vi "Get Path Commands.vi"(1 "Commands Raw Data":string) -> (0 "Array of Commands":T1(array[cluster]))   [LabVIEW 2011]
doc: "This VI takes in raw path data and outputs an array of all the commands found."
uses:
  <vilib>/Utility/error.llb/whitespace.ctl
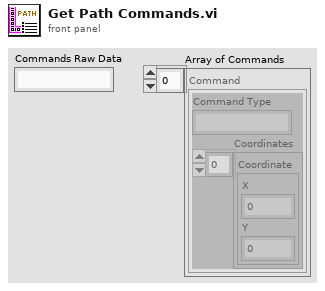
[diagram p1: front panel]
types:
  T1 = cluster{"Command Type":string, "Coordinates":cluster{"X":dbl, "Y":dbl}[]}[]
  T2 = typedef "whitespace.ctl" = u16
  T3 = cluster{"Commands Raw Data":string, cluster{dbl, dbl}[]}
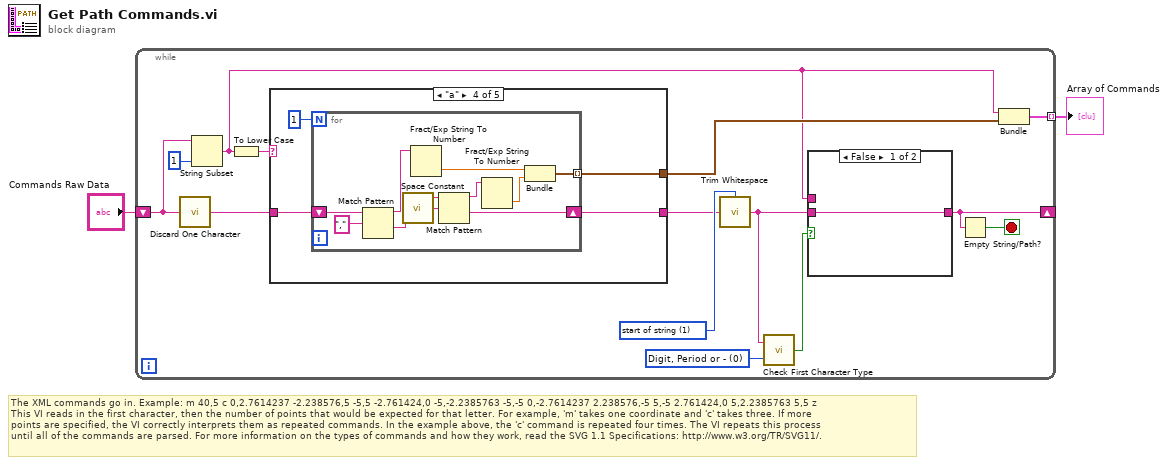
[diagram p0: block diagram]
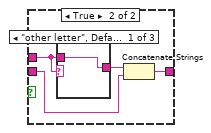
[diagram p2: hidden frame]
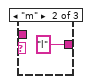
[diagram p3: hidden frame]
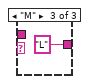
[diagram p4: hidden frame]
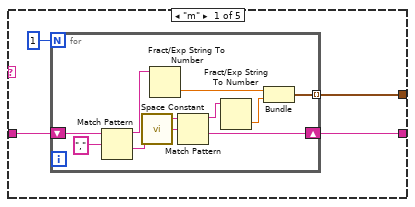
[diagram p5: hidden frame]
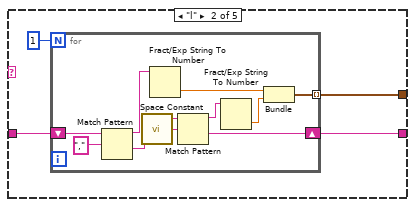
[diagram p6: hidden frame]
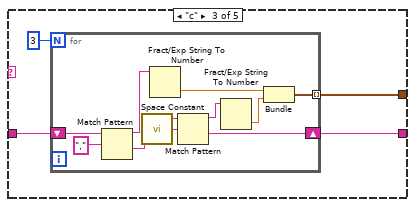
[diagram p7: hidden frame]
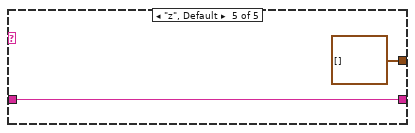
[diagram p8: hidden frame]
diagram:
  # "The XML commands go in. Example: m 40,5 c 0,2.7614237 -2.238576,5 -5,5 -2.761424,0 -5,-2.2385763 -5,-5 0,-2.7614237 2.238576,-5 5,-5 2.761424,0 5,2.2385763 5,5 z\nThis VI reads in the first character, then the number of points that would be expected for that letter. For example, 'm' takes one coordinate and 'c' takes three. If more\npoints are specified, the VI correctly interprets them as repeated commands. In the example above, the 'c' command is repeated four times. The VI repeats this process\nuntil all of the commands are parsed. For more information on the types of commands and how they work, read the SVG 1.1 Specifications: http://www.w3.org/TR/SVG11/."
  n1 = while {
    shift-right: [w3] -> _
    shift-left: "Commands Raw Data" -> [w5]
    tunnel: [w12] -> w2 mode=indexing
    stop <- w15 stop-if-true
    w9 = u16 0 items=["Digit, Period or -", "\"", "Character", "Space or Comma"] ("Type")
    w11 = T2 1 items=["both", "start of string", "end of string"] ("location (both)")
    n2 = call "Discard One Character.vi"("String"=w5) -> ("Remaining String"=w4:string)
    n3 = String Subset(string=w5, length (rest)=1 ("length (rest)")) -> (substring=w6:string)  [unwired: 1 in]
    n4 = To Lower Case(string=w6) -> (all lower case string=w13:string)
    n5 = case shown="\"a\"" w13 {
      tunnel: [w27 w41 w55 w69 cluster{dbl, dbl}[] []] -> w14
      tunnel: w4 -> [w26 w40 w54 w68 w81]
      tunnel: [w25 w39 w53 w67 w81] -> w10
      frame "m" {
        n6 = for {
          N: 1 -> [_]
          tunnel: [w30] -> w27 mode=indexing
          shift-right: [w29] -> w25
          shift-left: w26 -> [w37]
          n7 = Match Pattern(string=w37, regular expression=",") -> (before substring=w36:string, after substring=w35:string)  [unwired: 1 in, 2 out]
          n8 = call <vilib>:"Space Constant.vi"() -> ("String"=w34:string)
          n9 = Fract/Exp String To Number(string=w36) -> (number=w31:dbl)  [unwired: 3 in, 1 out]
          n10 = Match Pattern(string=w35, regular expression=w34) -> (before substring=w33:string, after substring=w29:string)  [unwired: 1 in, 2 out]
          n11 = Fract/Exp String To Number(string=w33) -> (number=w32:dbl)  [unwired: 3 in, 1 out]
          n12 = Bundle(w31, w32) -> (w30:cluster{dbl, dbl})  [unwired: 1 in]
        }
      }
      frame "l" {
        n13 = for {
          N: 1 -> [_]
          tunnel: [w44] -> w41 mode=indexing
          shift-right: [w43] -> w39
          shift-left: w40 -> [w51]
          n14 = Match Pattern(string=w51, regular expression=",") -> (before substring=w50:string, after substring=w49:string)  [unwired: 1 in, 2 out]
          n15 = call <vilib>:"Space Constant.vi"() -> ("String"=w48:string)
          n16 = Fract/Exp String To Number(string=w50) -> (number=w45:dbl)  [unwired: 3 in, 1 out]
          n17 = Match Pattern(string=w49, regular expression=w48) -> (before substring=w47:string, after substring=w43:string)  [unwired: 1 in, 2 out]
          n18 = Fract/Exp String To Number(string=w47) -> (number=w46:dbl)  [unwired: 3 in, 1 out]
          n19 = Bundle(w45, w46) -> (w44:cluster{dbl, dbl})  [unwired: 1 in]
        }
      }
      frame "c" {
        n20 = for {
          N: 3 -> [_]
          tunnel: [w58] -> w55 mode=indexing
          shift-right: [w57] -> w53
          shift-left: w54 -> [w65]
          n21 = Match Pattern(string=w65, regular expression=",") -> (before substring=w64:string, after substring=w63:string)  [unwired: 1 in, 2 out]
          n22 = call <vilib>:"Space Constant.vi"() -> ("String"=w62:string)
          n23 = Fract/Exp String To Number(string=w64) -> (number=w59:dbl)  [unwired: 3 in, 1 out]
          n24 = Match Pattern(string=w63, regular expression=w62) -> (before substring=w61:string, after substring=w57:string)  [unwired: 1 in, 2 out]
          n25 = Fract/Exp String To Number(string=w61) -> (number=w60:dbl)  [unwired: 3 in, 1 out]
          n26 = Bundle(w59, w60) -> (w58:cluster{dbl, dbl})  [unwired: 1 in]
        }
      }
      frame "a" {
        n27 = for {
          N: 1 -> [_]
          tunnel: [w72] -> w69 mode=indexing
          shift-right: [w71] -> w67
          shift-left: w68 -> [w79]
          n28 = Match Pattern(string=w79, regular expression=",") -> (before substring=w78:string, after substring=w77:string)  [unwired: 1 in, 2 out]
          n29 = call <vilib>:"Space Constant.vi"() -> ("String"=w76:string)
          n30 = Fract/Exp String To Number(string=w78) -> (number=w73:dbl)  [unwired: 3 in, 1 out]
          n31 = Match Pattern(string=w77, regular expression=w76) -> (before substring=w75:string, after substring=w71:string)  [unwired: 1 in, 2 out]
          n32 = Fract/Exp String To Number(string=w75) -> (number=w74:dbl)  [unwired: 3 in, 1 out]
          n33 = Bundle(w73, w74) -> (w72:cluster{dbl, dbl})  [unwired: 1 in]
        }
      }
      frame "z", Default {
      }
    }
    n34 = call <vilib>:"Trim Whitespace.vi"("string"=w10, "location (both)"=w11) -> ("trimmed string"=w7:string)
    n35 = call "Check First Character Type.vi"("Type"=w9, "Character"=w7) -> ("True/False"=w8:bool)
    n36 = case shown="False" w8 {
      tunnel: w7 -> [w17 w19]
      tunnel: w6 -> [_ w21]
      tunnel: [w17 w18] -> w3
      frame False {
      }
      frame True {
        n37 = case shown="\"other letter\", Default" w21 {
          tunnel: w21 -> [w22 _ _]
          tunnel: [w22 "l" "L"] -> w20
          frame "other letter", Default {
          }
          frame "m" {
          }
          frame "M" {
          }
        }
        n38 = Concatenate Strings(w20, w19) -> (w18:string)
      }
    }
    n39 = Empty String/Path?(string/path=w3) -> (empty?=w15:bool)
    n40 = Bundle("Commands Raw Data"=w6, w14) -> (w12:T3)  [unwired: 1 in]
  }
  "Array of Commands" <- w2
